vi "Read Record.vi"(8 "error in (no error)":errorcluster, 11 "Simulated Configuration Database Actor in":refnum<class "Sim Configuration Database Actor.lvclass">) -> (0 "error out":errorcluster, 3 "Simulated Configuration Database Actor out":refnum<class "Sim Configuration Database Actor.lvclass">)   [LabVIEW 2019, in "Sim Configuration Database Actor.lvlib" / "Sim Configuration Database Actor.lvclass"]
uses:
  Sim Configuration Database Actor.lvclass
  C:/Program Files (x86)/National Instruments/LabVIEW 2019/vi.lib/ActorFramework/Actor/Actor.lvclass
  <vilib>/ActorFramework/Actor/Actor.lvclass/Actor.ctl
  Sim Configuration Database Actor.lvclass/Sim Configuration Database Actor.ctl
  Car Wash Controller Actor/Car Wash Controller Actor Messages/Get Records Msg/Get Records Msg.lvclass/Get Records Msg.ctl
  <vilib>/ActorFramework/Message Enqueuer/Message Enqueuer.lvclass/Message Enqueuer.ctl
  <vilib>/ActorFramework/Message Enqueuer/Enqueue.vi
  Car Wash Controller Actor/Car Wash Controller Actor Messages/Get Records Msg/Get Records Msg.lvclass
  C:/Program Files (x86)/National Instruments/LabVIEW 2019/vi.lib/ActorFramework/Message/Message.lvclass
  <vilib>/ActorFramework/Message Priority Queue/Priority Enqueue.vi
  <vilib>/ActorFramework/Actor/Actor.lvclass
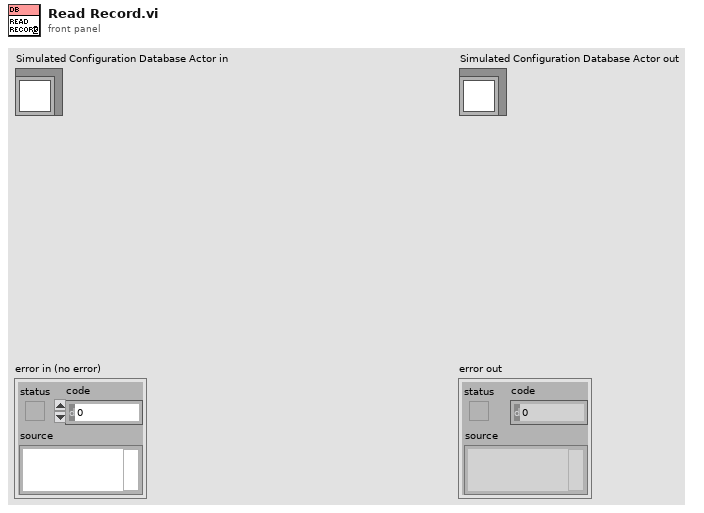
[diagram p1: front panel]
types:
  T1 = typedef "Sim Configuration Database Actor.lvlib/Sim Configuration Database Actor.lvclass/Records.ctl" = cluster{"Wash Step":string, "Station":string, "Step Duration":u32}
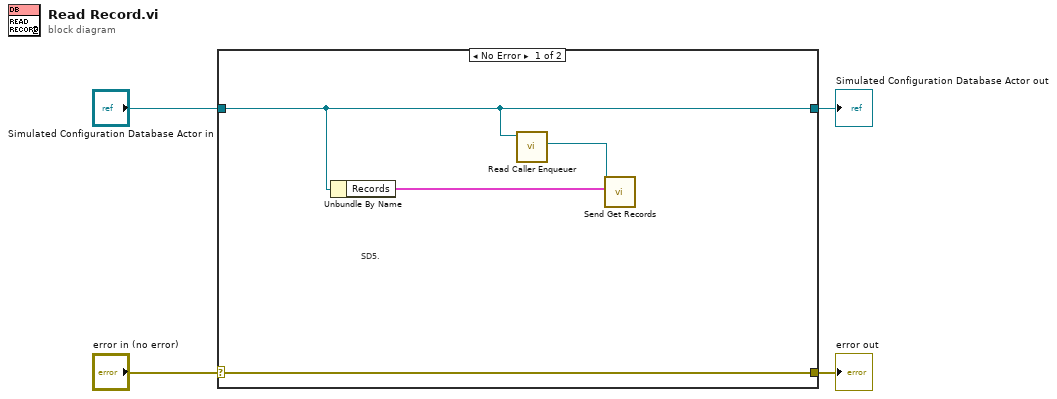
[diagram p0: block diagram]
diagram:
  n1 = case shown="No Error" "error in (no error)" {
    selector: "error in (no error)" -> [w8 w10]
    tunnel: [w8 w10] -> w3
    tunnel: [w7 w9] -> w1
    tunnel: "Simulated Configuration Database Actor in" -> [w7 w9]
    frame No Error {
      # "SD5."
      n2 = Unbundle By Name(w7) -> ("Records"=w5:T1)
      n3 = call <vilib>:"Read Caller Enqueuer.vi"("Actor"=w7) -> ("Caller Enqueuer"=w6:refnum<class "Message Enqueuer.lvclass">)  [unwired: 10 in]
      n4 = call "Send Get Records.vi"("Records"=w5, "Message Enqueuer"=w6) -> ()  [unwired: 8 in, 2 out]
    }
    frame Error {
    }
  }
  "error out" <- w3
  "Simulated Configuration Database Actor out" <- w1
